vi "solar_voy TCP Process.vi"(6 "Instance":i32, 8 "IP Address":string, 9 "Port":u16, 10 "Setup":T1, 11 "Voyager Refnum":T2) -> ()   [LabVIEW 2018]
doc: "This is the TCP read process launched by Voyager."
uses:
  solar_voy_ctl Voyager Refnum.ctl
  solar_voy_ctl Port Setup.ctl
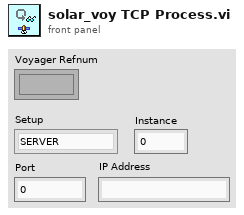
[diagram p1: front panel]
types:
  T1 = typedef "solar_voy_ctl Port Setup.ctl" = enum8{"SERVER", "CLIENT", "SERVER_CMD", "SERVER_TLM"}
  T2 = typedef "solar_voy_ctl Voyager Refnum.ctl" = refnum<k1>
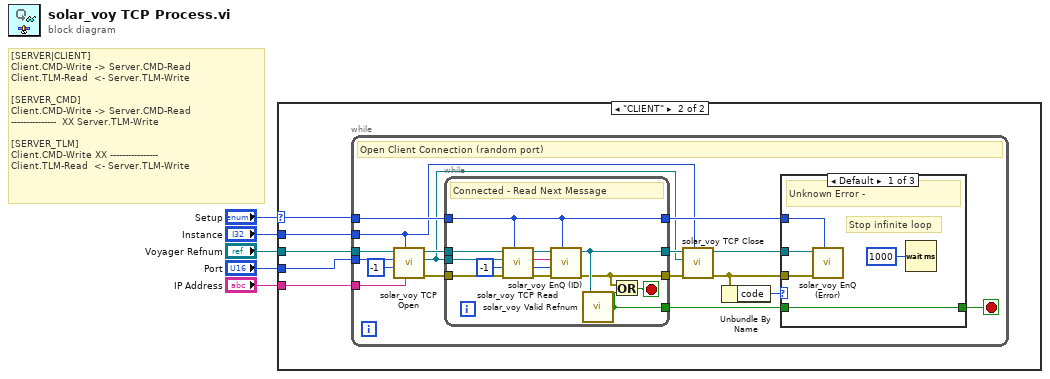
[diagram p0: block diagram]
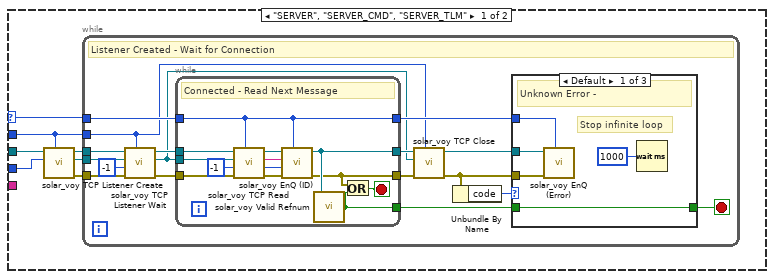
[diagram p2: hidden frame]
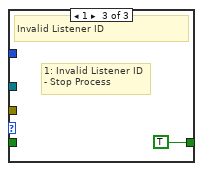
[diagram p4: hidden frame]
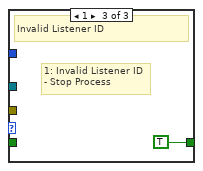
[diagram p6: hidden frame]
diagram:
  # "[SERVER|CLIENT]\nClient.CMD-Write -> Server.CMD-Read\nClient.TLM-Read  <- Server.TLM-Write\n\n[SERVER_CMD]\nClient.CMD-Write -> Server.CMD-Read\n---------------  XX Server.TLM-Write\n\n[SERVER_TLM]\nClient.CMD-Write XX ----------------\nClient.TLM-Read  <- Server.TLM-Write"
  n1 = case shown="\"CLIENT\"" "Setup" {
    selector: "Setup" -> [w6 w53]
    tunnel: "Voyager Refnum" -> [w12 w52]
    tunnel: "Port" -> [w8 w51]
    tunnel: "Instance" -> [w7 w54]
    tunnel: "IP Address" -> [_ w50]
    frame "SERVER", "SERVER_CMD", "SERVER_TLM" {
      n2 = call "solar_voy TCP Listener Create.vi"("Instance in"=w7, "Port"=w8, "Voyager Refnum in"=w12) -> ("error out"=w11:errorcluster, "Listener ID"=w10:refnum<k5>, "Voyager Refnum out"=w9:T2)  [unwired: 6 in]
      n3 = while {
        tunnel: w11 -> [w29]
        tunnel: w10 -> [w25]
        tunnel: w9 -> [w24]
        tunnel: w7 -> [w13]
        tunnel: w6 -> [w22]
        stop <- w26 stop-if-true
        # "Listener Created - Wait for Connection"
        n4 = call "solar_voy TCP Listener Wait.vi"("Instance"=w13, "error in (no error)"=w29, "timeout ms (-1)"=-1, "Listener ID"=w25, "Voyager Refnum in"=w24) -> ("error out"=w28:errorcluster, "Connection ID"=w16:refnum<k5>, "Voyager Refnum out"=w23:T2)  [unwired: 4 in]
        n5 = while {
          tunnel: w28 -> [w42]
          tunnel: w16 -> [w38]
          tunnel: [w33] -> w18
          tunnel: [w34] -> w17
          tunnel: w23 -> [w39]
          tunnel: w22 -> [w30]
          tunnel: [w31] -> w20
          tunnel: [w30] -> w19
          stop <- w32 stop-if-true
          # "Connected - Read Next Message"
          n6 = call "solar_voy TCP Read.vi"("Setup"=w30, "error in (no error)"=w42, "timeout ms (-1)"=-1, "Connection ID"=w38, "Voyager Refnum in"=w39) -> ("error out"=w41:errorcluster, "ID"=w35:u16, "TCP Data"=w40:string, "Voyager Refnum out"=w36:T2)  [unwired: 3 in]
          n7 = call "solar_voy EnQ (ID).vi"("Setup"=w30, "error in (no error)"=w41, "ID"=w35, "TCP Data"=w40, "Voyager Refnum in"=w36) -> ("error out"=w33:errorcluster, "Voyager Refnum out"=w34:T2)  [unwired: 5 in]
          n8 = call "solar_voy Valid Refnum.vi"("Voyager Refnum"=w34) -> ("Invalid Refnum?"=w31:bool)
          n9 = Or(x=w33, y=w31) -> (x .or. y?=w32:bool)
        }
        n10 = call "solar_voy TCP Close.vi"("Instance"=w13, "error in (no error)"=w18, "Connection ID"=w16, "Voyager Refnum in"=w17) -> ("error out"=w15:errorcluster, "Voyager Refnum out"=w14:T2)  [unwired: 6 in]
        n11 = Unbundle By Name(w15) -> ("code"=w27:i32)
        n12 = case shown="Default" w27 {
          tunnel: [w46 w48 TRUE ("Invalid Refnum?")] -> w26
          tunnel: w15 -> [w44 _ _]
          tunnel: w14 -> [w45 _ _]
          tunnel: w20 -> [w46 w48 _]
          tunnel: w19 -> [w43 _ _]
          frame Default {
            # "Stop infinite loop"
            # "Unknown Error -"
            n13 = call "solar_voy EnQ (Error).vi"("Setup"=w43, "error in (no error)"=w44, "Voyager Refnum in"=w45) -> ()  [unwired: 7 in, 2 out]
            n14 = Wait (ms)(milliseconds to wait=u32 1000) -> ()  [unwired: 1 out]
          }
          frame 56, 66 {
            # "56: Connection Timed Out\n66: Connection Closed"
            # "Errors to Ignore"
          }
          frame 1 {
            # "1: Invalid Listener ID\n- Stop Process"
            # "Invalid Listener ID"
          }
        }
      }
    }
    frame "CLIENT" {
      n15 = while {
        tunnel: w54 -> [w57]
        tunnel: w53 -> [w69]
        tunnel: w52 -> [w59]
        tunnel: w51 -> [w56]
        tunnel: w50 -> [w55]
        stop <- w70 stop-if-true
        # "Open Client Connection (random port)"
        n16 = call "solar_voy TCP Open.vi"("IP Address"=w55, "Instance"=w57, "timeout ms (-1)"=-1, "Port"=w56, "Voyager Refnum in"=w59) -> ("error out"=w62:errorcluster, "Connection ID"=w58:refnum<k5>, "Voyager Refnum out"=w60:T2)  [unwired: 4 in]
        n17 = while {
          tunnel: w62 -> [w84]
          tunnel: w58 -> [w80]
          tunnel: [w75] -> w66
          tunnel: [w76] -> w65
          tunnel: w60 -> [w81]
          tunnel: w69 -> [w72]
          tunnel: [w73] -> w68
          tunnel: [w72] -> w67
          stop <- w74 stop-if-true
          # "Connected - Read Next Message"
          n18 = call "solar_voy TCP Read.vi"("Setup"=w72, "error in (no error)"=w84, "timeout ms (-1)"=-1, "Connection ID"=w80, "Voyager Refnum in"=w81) -> ("error out"=w83:errorcluster, "ID"=w77:u16, "TCP Data"=w82:string, "Voyager Refnum out"=w78:T2)  [unwired: 3 in]
          n19 = call "solar_voy EnQ (ID).vi"("Setup"=w72, "error in (no error)"=w83, "ID"=w77, "TCP Data"=w82, "Voyager Refnum in"=w78) -> ("error out"=w75:errorcluster, "Voyager Refnum out"=w76:T2)  [unwired: 5 in]
          n20 = call "solar_voy Valid Refnum.vi"("Voyager Refnum"=w76) -> ("Invalid Refnum?"=w73:bool)
          n21 = Or(x=w75, y=w73) -> (x .or. y?=w74:bool)
        }
        n22 = call "solar_voy TCP Close.vi"("Instance"=w57, "error in (no error)"=w66, "Connection ID"=w58, "Voyager Refnum in"=w65) -> ("error out"=w64:errorcluster, "Voyager Refnum out"=w63:T2)  [unwired: 6 in]
        n23 = Unbundle By Name(w64) -> ("code"=w71:i32)
        n24 = case shown="Default" w71 {
          tunnel: [w88 w90 TRUE ("Invalid Refnum?")] -> w70
          tunnel: w64 -> [w86 _ _]
          tunnel: w63 -> [w87 _ _]
          tunnel: w68 -> [w88 w90 _]
          tunnel: w67 -> [w85 _ _]
          frame Default {
            # "Stop infinite loop"
            # "Unknown Error -"
            n25 = call "solar_voy EnQ (Error).vi"("Setup"=w85, "error in (no error)"=w86, "Voyager Refnum in"=w87) -> ()  [unwired: 7 in, 2 out]
            n26 = Wait (ms)(milliseconds to wait=u32 1000) -> ()  [unwired: 1 out]
          }
          frame 56, 63, 66 {
            # "56: Connection Timed Out\n63: Refused by server\n66: Connection Closed"
            # "Errors to Ignore"
          }
          frame 1 {
            # "1: Invalid Listener ID\n- Stop Process"
            # "Invalid Listener ID"
          }
        }
      }
    }
  }
